vi "AC Output Frequency Test.vi"(7 "Test Socket (0)":i32, 11 "Scope in":string) -> (0 "error out":errorcluster, 2 "Waveform Data":dbl[](array[numeric]), 3 "Frequency":dbl)   [LabVIEW 2025]
doc: "Measures the frequency of the AC signal. Before calling this VI, ensure that the input signal is set for the battery pin."
uses:
  <vilib>/measure/matone.llb/Extract Single Tone Information 1 Chan.vi
  Program Files (x86)/National Instruments/LabVIEW 2024/Instr.lib/Driver Simulation/Oscilloscope.lvlib
  <vilib>/measure/NI_MAPro.lvlib
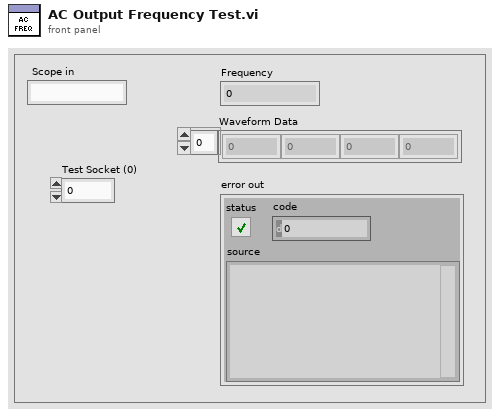
[diagram p1: front panel]
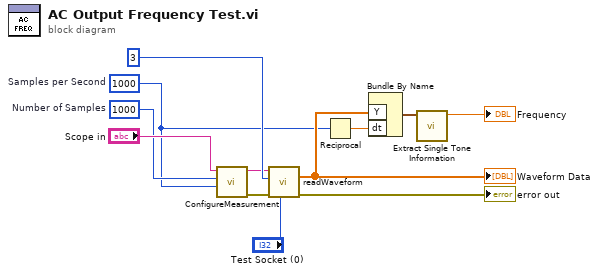
[diagram p0: block diagram]
diagram:
  w2 = 1000  # Samples per Second
  w6 = 1000  # Number of Samples
  n1 = call "ConfigureMeasurement.vi"("Samples Per Second"=w2, "Number of Samples"=w6, "Scope in"="Scope in") -> ("error out"=w9:errorcluster, "Scope out"=w10:string)  [unwired: 7 in]
  n2 = call "readWaveform.vi"("Test Socket (0)"="Test Socket (0)", "error in (no error)"=w9, "Channel"=3 ("Scope Channel"), "Scope in"=w10) -> ("error out"=→"error out":errorcluster, "Result"=w3:dbl[])  [unwired: 5 in, 1 out]
  "Waveform Data" <- w3
  n3 = Reciprocal(x=w2) -> (1/x=w5:dbl)
  n4 = Bundle By Name("Y"=w3, "dt"=w5) -> (w4:waveform(dbl))  [unwired: 1 in]
  n5 = call-poly <vilib>:"Extract Single Tone Information.vi"("time signal in"=w4) -> ("detected frequency"=→"Frequency":dbl)  [unwired: 5 in, 5 out]
